vi "Read Lock-in configuration.vi"(8 "error in (no error)":errorcluster, 11 "Lock-in Driver in":refnum<class "Lock-in Driver.lvclass">) -> (0 "error out":errorcluster, 2 "Configuration":T1={"Frequency"=0.0, "Time constant"=0.0, "Synchronous"=FALSE, "Channels"=[1]} {"Time constant" min=0.000263 max=0.53687 format="%#_8ps"; "Frequency" format="%#_6pHz"}, 3 "Lock-in Driver out":refnum<class "Lock-in Driver.lvclass">)   [LabVIEW 2019, in "Lock-in Driver.lvclass"]
uses:
  Lock-in Driver.lvclass
  C:/GitHub/NHMFL_Core/Libraries/Instruments/Instrument Driver/Instrument Driver.lvclass
  Lock-in Configuration.ctl
  Read User configuration.vi
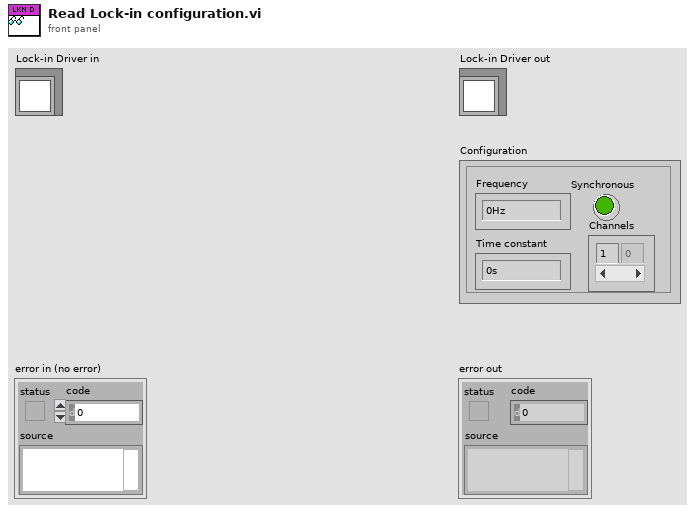
[diagram p1: front panel]
types:
  T1 = typedef "Lock-in Configuration.ctl" = cluster{"Frequency":dbl, "Time constant":dbl, "Synchronous":bool, "Channels":i32[]}
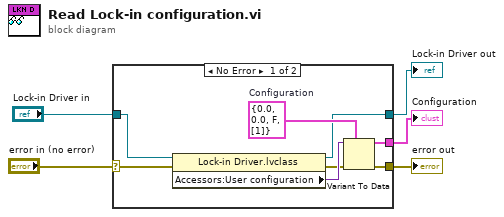
[diagram p0: block diagram]
diagram:
  n1 = case shown="No Error" "error in (no error)" {
    selector: "error in (no error)" -> [w6 w14]
    tunnel: [w13 w14] -> w4
    tunnel: [w8 w15] -> w2
    tunnel: "Lock-in Driver in" -> [w9 w15]
    tunnel: [w7 _] -> w1
    frame No Error {
      w11 = T1 {"Frequency"=0.0, "Time constant"=0.0, "Synchronous"=FALSE, "Channels"=[1]}  # Configuration
      n2 = property class="Lock-in Driver.lvclass"(reference=w9, error in=w6) -> (reference out=w8:refnum<class "Lock-in Driver.lvclass">, error out=w10:errorcluster, "Accessors:User configuration"=w12:variant)
      n3 = Variant To Data(error in=w10, type=w11, Variant=w12) -> (data=w7:T1, error out=w13:errorcluster)
    }
    frame Error {
    }
  }
  "error out" <- w4
  "Lock-in Driver out" <- w2
  "Configuration" <- w1
